vi "Read Offline Data.vi"(8 "Error In":errorcluster) -> (0 "Error Out":errorcluster)   [LabVIEW 2014, in "Aquisicao de Dados.lvlib"]
uses:
  Aquisicao de Dados.lvlib
panel:
  out "Canal 1":waveform(dbl)(graph)
  out "Canal 0":waveform(dbl)(graph)
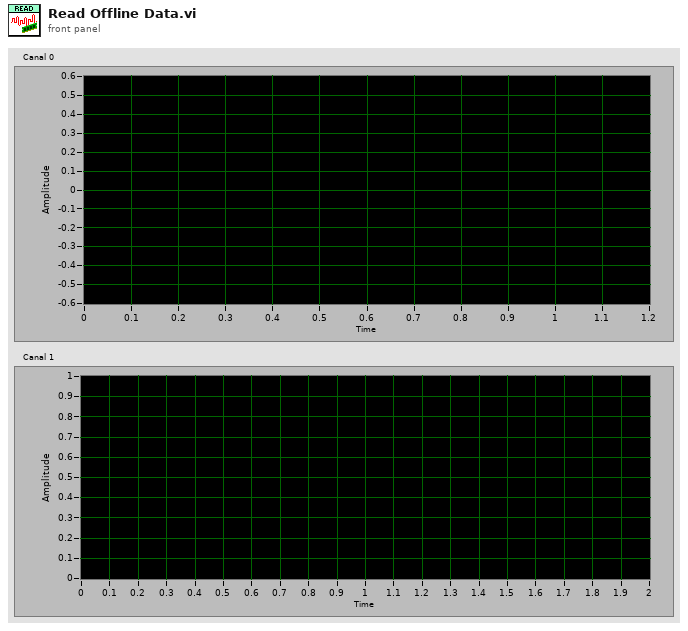
[diagram p1: front panel]
types:
  T1 = enum32{".WAV File", "LTSpice Simulation", "Microphone", "MultiSim Simulation", "Serial Port"}
  T2 = typedef "Aquisicao de Dados.lvlib/_ACC_DATA_ Config DAta State.ctl" = cluster{"_RAW_ Traces":cluster{"Trace Name":string, "Trace Type":string, "Trace Raw Data":dbl[], "Trace Waveform":waveform(dbl)}[], "_WAV_ Traces":waveform(dbl)[], "_MIC_ Config":cluster{"task ID":T3, "Data Chunk Size":i32, "Num Channels":i32, "Resolution":i32, "Sampling Frequency":dbl, "device ID":u32, "Num Chunks":i32}, "_LVM_ Traces":cluster{"Trace Name":string, "Trace Type":string, "Trace Raw Data":dbl[], "Trace Waveform":waveform(dbl)}[]}
  T3 = typedef "Sound Input Task ID.ctl" = u32
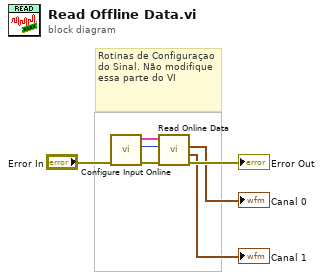
[diagram p0: block diagram]
diagram:
  # "Rotinas de Configuraçao do Sinal. Não modifique essa parte do VI"
  n1 = call "Configure Input Online.vi"("Error In"="Error In") -> ("Error Out"=w7:errorcluster, "Metodo de Entrada"=w5:T1, "Config Out"=w3:T2)  [unwired: 8 in]
  n2 = call "Read Online Data.vi"("Error In"=w7, "Metodo de Entrada"=w5, "Config Out"=w3) -> ("Error Out"=→"Error Out":errorcluster, "Channel 1"=→"Canal 1":waveform(dbl), "Channel 0"=→"Canal 0":waveform(dbl))  [unwired: 6 in]
